vi "Write Active.vi"(7 "SPI CS":refnum<class "SPI CS.lvclass">, 8 "error in (no error)":errorcluster, 10 "Active":bool, 11 "Session In":refnum<class "Session.lvclass">) -> (0 "error out":errorcluster, 3 "Session Out":refnum<class "Session.lvclass">)   [LabVIEW 2024, in "CTI.lvlib" / "SPI CS.lvclass"]
uses:
  SPI CS.lvclass
  Session/Session.lvclass
  GPIO Number.ctl
  SPI CS.lvclass/SPI CS.ctl
  CTI.lvlib
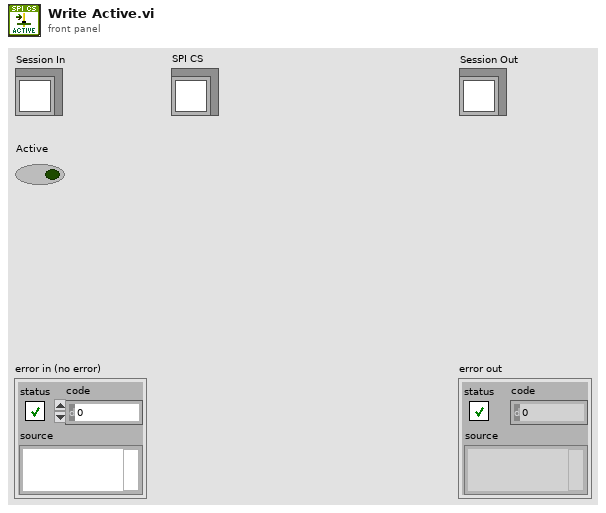
[diagram p1: front panel]
types:
  T1 = typedef "CTI.lvlib/GPIO Number.ctl" = i8
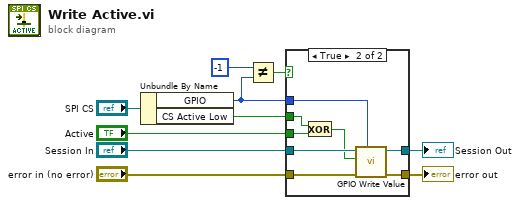
[diagram p0: block diagram]
diagram:
  n1 = Unbundle By Name("SPI CS") -> ("GPIO"=w3:T1, "CS Active Low"=w8:bool)
  n2 = Not Equal?(x=T1 -1, y=w3) -> (x != y?=w2:bool)
  n3 = case shown="True" w2 {
    tunnel: "Active" -> [_ w20]
    tunnel: w8 -> [_ w19]
    tunnel: "Session In" -> [w12 w18]
    tunnel: "error in (no error)" -> [w11 w17]
    tunnel: [w11 w16] -> w5
    tunnel: [w12 w14] -> w4
    tunnel: w3 -> [_ w13]
    frame False {
    }
    frame True {
      n4 = Exclusive Or(1:w20, 2:w19) -> (0:w15:bool)
      n5 = call "GPIO Write Value.vi"("GPIO #"=w13, "error in (no error)"=w17, "Value"=w15, "Session in"=w18) -> ("error out"=w16:errorcluster, "Session out"=w14:refnum<class "Session.lvclass">)  [unwired: 6 in]
    }
  }
  "error out" <- w5
  "Session Out" <- w4
